vi "Autonomous Independent.vi"() -> ()   [LabVIEW 2011]
doc: "This VI is called when autonomous begins, and will automatically be terminated when autonomous ends. You can carry out timed or sensor driven robot movement independently without needing to return to the caller."
uses:
  Robot Global Data.vi
  <vilib>/addons/control/pid/pid.llb/PID (DBL).vi
  <vilib>/addons/control/pid/NI_PID_pid.lvlib
  <vilib>/Analysis/NI_AALBase.lvlib
panel:
  in  "Gains Left":T1={"proportional gain (Kc)"=0.01, "integral time (Ti, min)"=0.0, "derivative time (Td, min)"=0.001}
  in  "Gains Right":T1={"proportional gain (Kc)"=0.01, "integral time (Ti, min)"=0.0, "derivative time (Td, min)"=0.001}
  out "Right Output":dbl(graph)
  out "Right Encoder":dbl(graph)
  out "Left Enoder":dbl(graph)
  out "Left Output":dbl(graph)
  out "Autonomous Switch Value":dbl
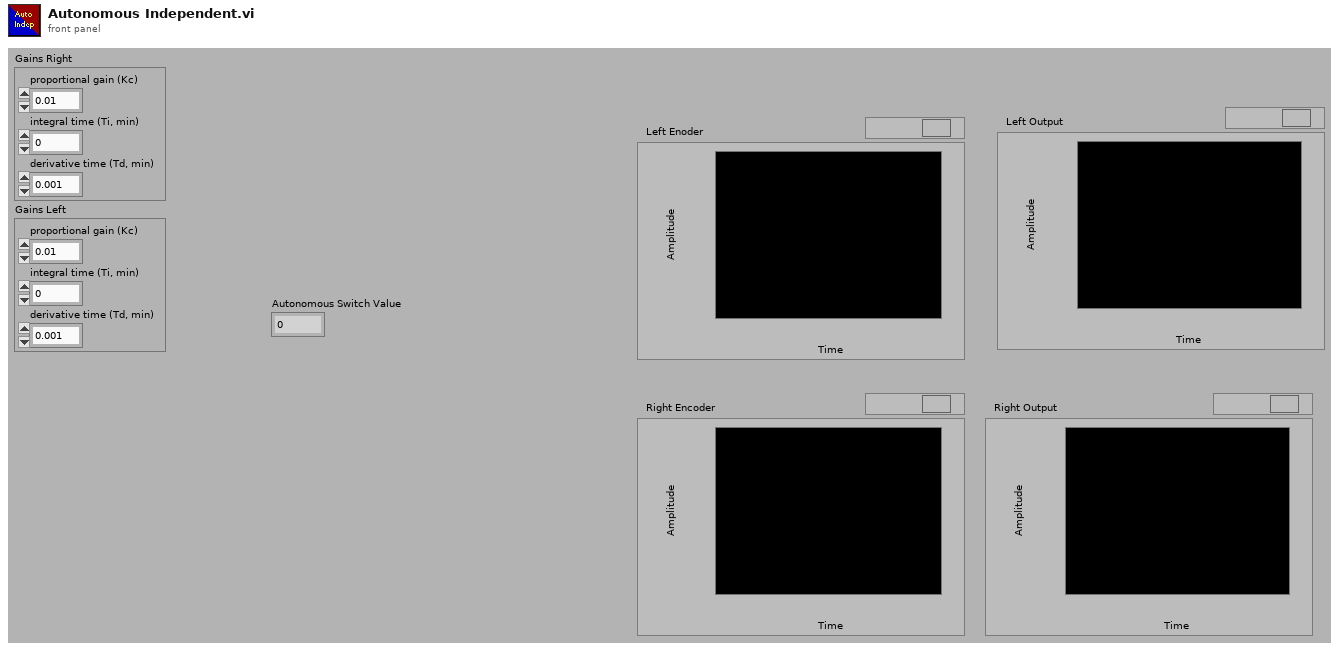
[diagram p1: front panel]
types:
  T1 = cluster{"proportional gain (Kc)":dbl, "integral time (Ti, min)":dbl, "derivative time (Td, min)":dbl}
  T2 = typedef "WPI_JoystickDevRef.ctl" = cluster{"Device":T3}
  T3 = typedef "WPI_JoystickDeviceEnum.ctl" = enum16{"USB 1", "USB 2", "USB 3", "USB 4", "Kinect 1", "Kinect 2"}
  T4 = typedef "WPI_DigitalInputDevRef.ctl" = cluster{"DevStatus":errorcluster, "DIO Channel":T5, "Digital Module":T6}
  T5 = typedef "FPGA_DIOChannel.ctl" = enum8{"DIO 1", "DIO 2", "DIO 3", "DIO 4", "DIO 5", "DIO 6", "DIO 7", "DIO 8", "DIO 9", "DIO 10", "DIO 11", "DIO 12", "DIO 13", "DIO 14", "Invalid"}
  T6 = typedef "FPGA_TypedefDigitalModule.ctl" = enum16{"Digital Module 1", "Digital Module 2"}
  T7 = cluster{"axis 1 (x)":dbl, "axis 2 (y)":dbl, "axis 3 (throttle)":dbl, "axis 4":dbl, "axis 5":dbl, "axis 6":dbl}
  T8 = enum16{"Shoot", "Load", "Arm", "Nothing", "Reverse", "ShootAll"}
  T9 = typedef "WPI_RobotDriveDevRef.ctl" = cluster{"DevStatus":errorcluster, "Motors[]":T10[], "Square Inputs":bool, "Max Output":dbl, "Isochronous":bool}
  T10 = typedef "WPI_MotorControlDeviceRef.ctl" = cluster{"DeviceStatus":errorcluster, "Type":enum16{"PWM", "CAN"}, "PWM":cluster{"Digital Module":T6, "PWM Channel":T11, "DeadBand":T12}, "CAN":cluster{"Device Number":u8, "Control Mode":T13, "Semaphore":T14, "Max Vout":dbl}, "Invert":bool, "TransformRef":T15, "InvTransformRef":T15}
  T11 = typedef "FPGA_DIOPWMChannel.ctl" = enum8{"PWM 1", "PWM 2", "PWM 3", "PWM 4", "PWM 5", "PWM 6", "PWM 7", "PWM 8", "PWM 9", "PWM 10", "Invalid"}
  T12 = typedef "WPI_PWMDeadband.ctl" = cluster{"Name":string, "maxPositivePwm":i32, "minPositivePwm":i32, "centerPwm":i32, "maxNegativePwm":i32, "minNegativePwm":i32, "angularRange":u16}
  T13 = typedef "WPI_CANJaguar_ControlMode.ctl" = enum8{"Percent VBus", "Current", "Speed", "Position", "Voltage"}
  T14 = typedef "Semaphore RefNum" = refnum<k1>
  T15 = typedef "WPI_PWMTransform_ConPane.ctl" = refnum<vi>
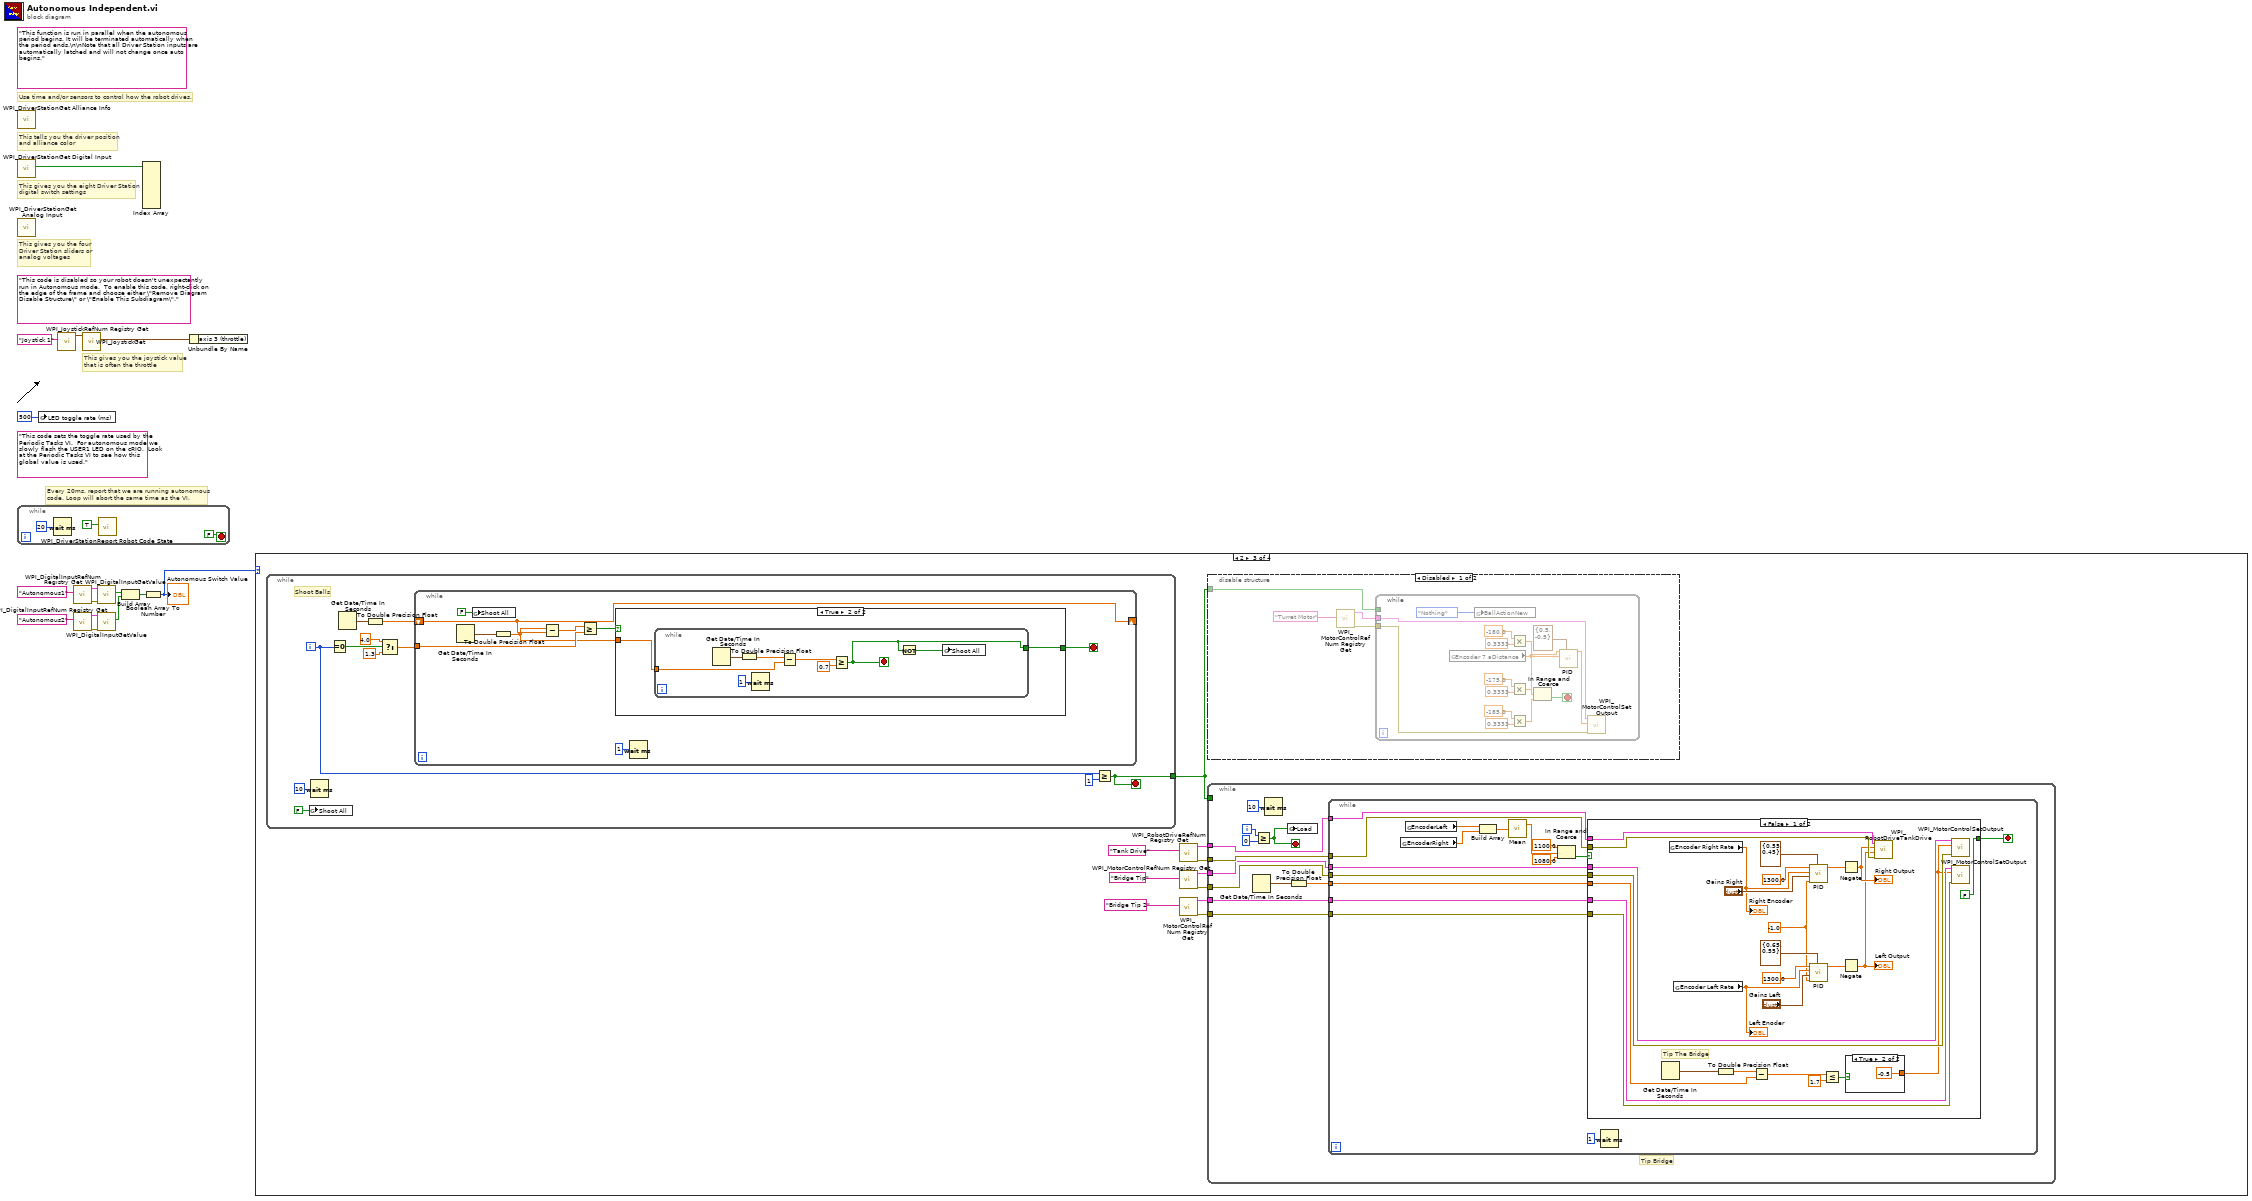
[diagram p0: block diagram]
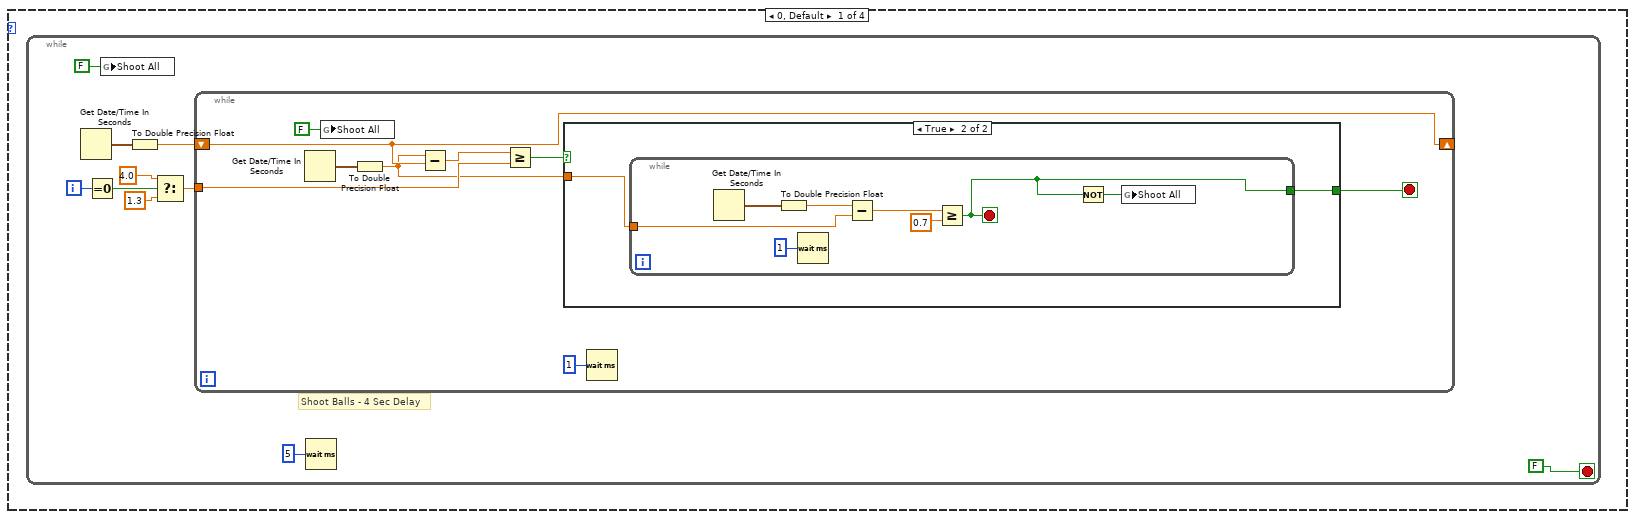
[diagram p2: hidden frame]
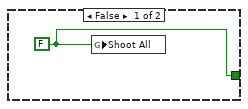
[diagram p3: hidden frame]
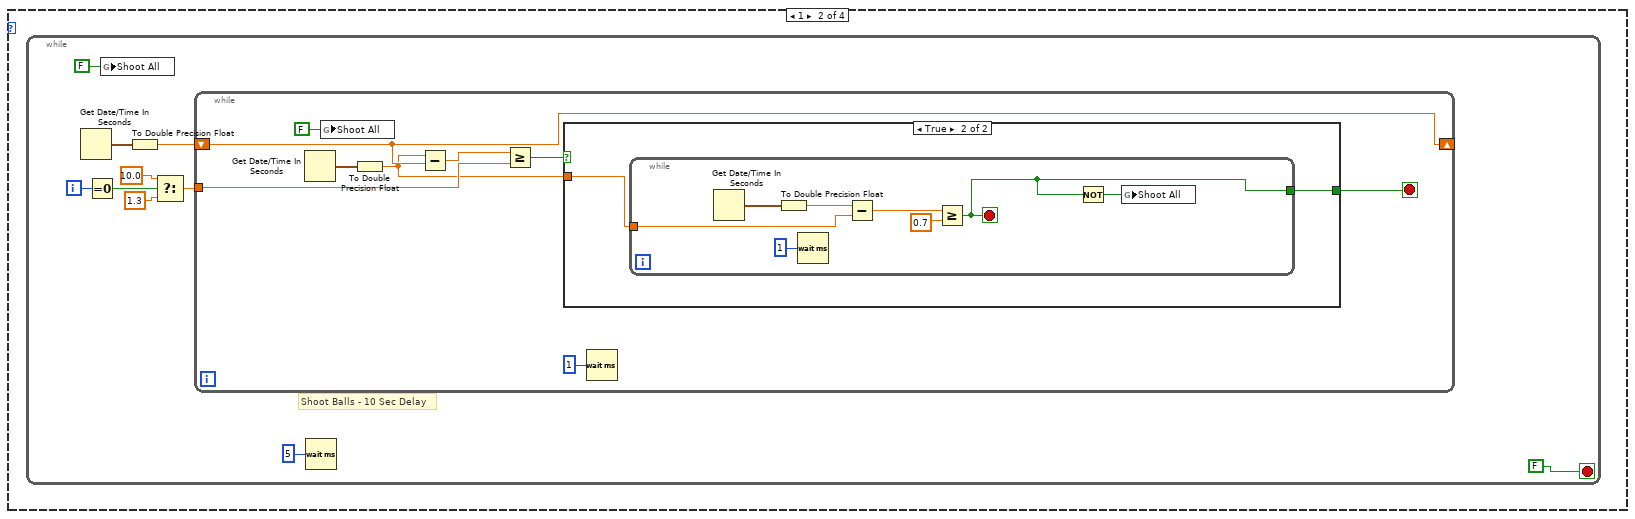
[diagram p4: hidden frame]
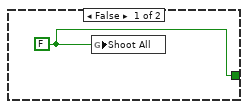
[diagram p5: hidden frame]
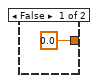
[diagram p7: hidden frame]
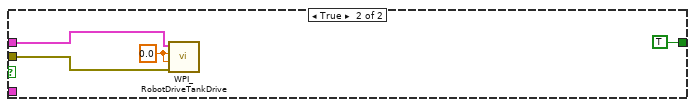
[diagram p8: hidden frame]
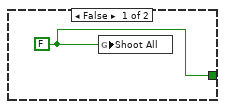
[diagram p9: hidden frame]
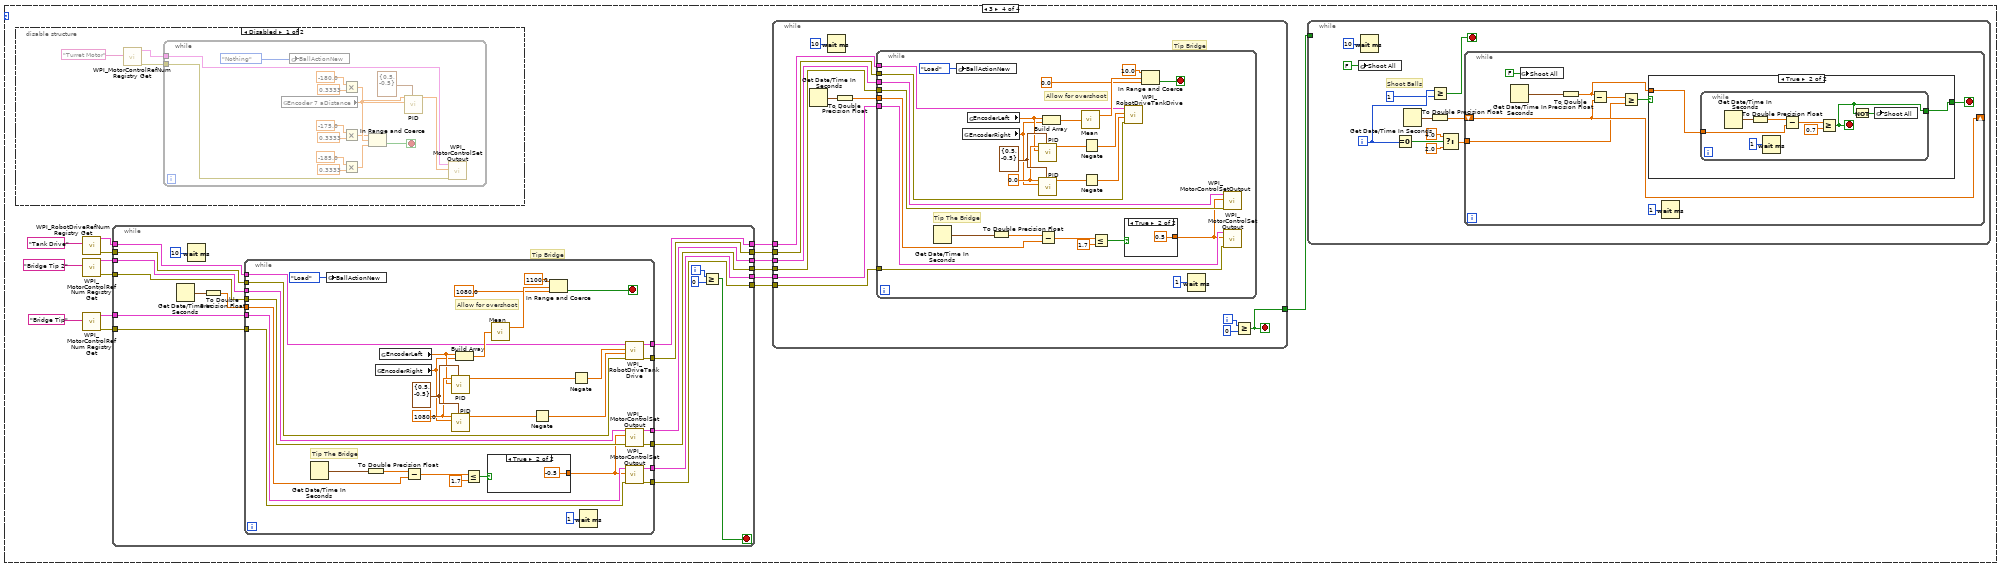
[diagram p10: hidden frame]
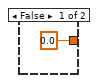
[diagram p11: hidden frame]
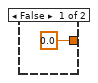
[diagram p13: hidden frame]
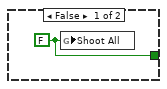
[diagram p14: hidden frame]
diagram:
  (unwired) "This code sets the toggle rate used by the Periodic Tasks VI.  For autonomous mode we slowly flash the USER1 LED on the cRIO.  Look at the Periodic Tasks VI to see how this global value is used."
  (unwired) "This code is disabled so your robot doesn't unexpectantly run in Autonomous mode.  To enable this code, right-click on the edge of the frame and choose either \"Remove Diagram Disable Structure\" or \"Enable This Subdiagram\"."
  (unwired) "This function is run in parallel when the autonomous period begins. It will be terminated automatically when the period ends.\n\nNote that all Driver Station inputs are automatically latched and will not change once auto begins."
  # "Every 20ms, report that we are running autonomous\ncode. Loop will abort the same time as the VI."
  # "This gives you the joystick value\nthat is often the throttle"
  # "Use time and/or sensors to control how the robot drives."
  # "This tells you the driver position\nand alliance color"
  # "This gives you the eight Driver Station\ndigital switch settings"
  # "This gives you the four\nDriver Station sliders or\nanalog voltages"
  n1 = call <vilib>:"WPI_DriverStationGet Alliance Info.vi"() -> ()  [unwired: 12 out]
  n2 = call <vilib>:"WPI_DriverStationGet Digital Input.vi"() -> ("Driver Station Digital Input (1-8)"=w15:bool[])  [unwired: 11 out]
  n3 = call <vilib>:"WPI_DriverStationGet Analog Input.vi"() -> ()  [unwired: 12 out]
  n4 = while {
    stop <- FALSE stop-if-true
    n5 = Wait (ms)(milliseconds to wait=u32 20) -> ()  [unwired: 1 out]
    n6 = call <vilib>:"WPI_DriverStationReport Robot Code State.vi"("Autonomous"=TRUE) -> ()  [unwired: 10 in, 1 out]
  }
  n7 = global write "Robot Global Data.vi" "LED toggle rate (ms)"(u32 500 ("LED ms toggle rate")) -> ()
  n8 = call <vilib>:"WPI_JoystickRefNum Registry Get.vi"("refnum name"="Joystick 1") -> ("JoystickDevRef"=w12:T2)  [unwired: 1 in, 9 out]
  n9 = call <vilib>:"WPI_DigitalInputRefNum Registry Get.vi"("refnum name"="Autonomous1") -> ("error out"=w8:errorcluster, "DigitalInputDevRef"=w7:T4)  [unwired: 9 in]
  n10 = call <vilib>:"WPI_DigitalInputRefNum Registry Get.vi"("refnum name"="Autonomous2") -> ("error out"=w5:errorcluster, "DigitalInputDevRef"=w6:T4)  [unwired: 9 in]
  n11 = call <vilib>:"WPI_JoystickGet.vi"("JoystickDevRef"=w12) -> ("Axes"=w13:T7)  [unwired: 1 in, 5 out]
  n12 = call <vilib>:"WPI_DigitalInputGetValue.vi"("error in (no error)"=w8, "DigitalInputDevRef"=w7) -> ("Value"=w9:bool)  [unwired: 7 in, 2 out]
  n13 = call <vilib>:"WPI_DigitalInputGetValue.vi"("error in (no error)"=w5, "DigitalInputDevRef"=w6) -> ("Value"=w10:bool)  [unwired: 7 in, 2 out]
  n14 = Build Array(w9, w10) -> (w2:bool[])
  n15 = Index Array(array=w15) -> ()  [unwired: 8 in, 8 out]
  n16 = Boolean Array To Number(Boolean array=w2) -> (number=w1:u32)
  "Autonomous Switch Value" <- w1
  n17 = Unbundle By Name(w13) -> ()  [unwired: 1 out]
  n18 = case shown="2" w1 {
    frame 0, Default {
      n19 = while {
        i -> [w24]
        stop <- FALSE stop-if-true
        # "Shoot Balls - 4 Sec Delay"
        n20 = Get Date/Time In Seconds() -> (seconds since 1Jan1904=w28:timestamp)
        n21 = Equal To 0?(x=w24) -> (x = 0?=w23:bool)
        n22 = global write "Robot Global Data.vi" "Shoot All"(FALSE ("Shoot All")) -> ()
        n23 = To Double Precision Float(number=w28) -> (double precision float=w27:dbl)
        n24 = Select(t=4.0, s=w23, f=1.3) -> (s? t:f=w22:dbl)
        n25 = while {
          shift-right: [w37] -> _
          shift-left: w27 -> [w37]
          tunnel: w22 -> [w35]
          stop <- w34 stop-if-true
          n26 = Get Date/Time In Seconds() -> (seconds since 1Jan1904=w33:timestamp)
          n27 = global write "Robot Global Data.vi" "Shoot All"(FALSE ("Shoot All")) -> ()
          n28 = To Double Precision Float(number=w33) -> (double precision float=w31:dbl)
          n29 = Subtract(x=w31, y=w37) -> (x-y=w32:dbl)
          n30 = Greater Or Equal?(x=w32, y=w35) -> (x >= y?=w30:bool)
          n31 = case shown="True" w30 {
            tunnel: [w38 w40] -> w34
            tunnel: w31 -> [_ w39]
            frame False {
              w38 = FALSE
              n32 = global write "Robot Global Data.vi" "Shoot All"(w38) -> ()
            }
            frame True {
              n33 = while {
                tunnel: w39 -> [w46]
                tunnel: [w41] -> w40
                stop <- w41 stop-if-true
                n34 = Get Date/Time In Seconds() -> (seconds since 1Jan1904=w48:timestamp)
                n35 = To Double Precision Float(number=w48) -> (double precision float=w47:dbl)
                n36 = Wait (ms)(milliseconds to wait=u32 1) -> ()  [unwired: 1 out]
                n37 = Subtract(x=w47, y=w46) -> (x-y=w45:dbl)
                n38 = Greater Or Equal?(x=w45, y=0.7) -> (x >= y?=w41:bool)
                n39 = Not(x=w41) -> (.not. x?=w42:bool)
                n40 = global write "Robot Global Data.vi" "Shoot All"(w42) -> ()
              }
            }
          }
          n41 = Wait (ms)(milliseconds to wait=u32 1) -> ()  [unwired: 1 out]
        }
        n42 = Wait (ms)(milliseconds to wait=u32 5) -> ()  [unwired: 1 out]
      }
    }
    frame 1 {
      n43 = while {
        i -> [w54]
        stop <- FALSE stop-if-true
        # "Shoot Balls - 10 Sec Delay"
        n44 = Get Date/Time In Seconds() -> (seconds since 1Jan1904=w58:timestamp)
        n45 = Equal To 0?(x=w54) -> (x = 0?=w53:bool)
        n46 = global write "Robot Global Data.vi" "Shoot All"(FALSE ("Shoot All")) -> ()
        n47 = To Double Precision Float(number=w58) -> (double precision float=w57:dbl)
        n48 = Select(t=10.0, s=w53, f=1.3) -> (s? t:f=w52:dbl)
        n49 = while {
          shift-right: [w67] -> _
          shift-left: w57 -> [w67]
          tunnel: w52 -> [w65]
          stop <- w64 stop-if-true
          n50 = Get Date/Time In Seconds() -> (seconds since 1Jan1904=w63:timestamp)
          n51 = global write "Robot Global Data.vi" "Shoot All"(FALSE ("Shoot All")) -> ()
          n52 = To Double Precision Float(number=w63) -> (double precision float=w61:dbl)
          n53 = Subtract(x=w61, y=w67) -> (x-y=w62:dbl)
          n54 = Greater Or Equal?(x=w62, y=w65) -> (x >= y?=w60:bool)
          n55 = case shown="True" w60 {
            tunnel: [w68 w70] -> w64
            tunnel: w61 -> [_ w69]
            frame False {
              w68 = FALSE
              n56 = global write "Robot Global Data.vi" "Shoot All"(w68) -> ()
            }
            frame True {
              n57 = while {
                tunnel: w69 -> [w76]
                tunnel: [w71] -> w70
                stop <- w71 stop-if-true
                n58 = Get Date/Time In Seconds() -> (seconds since 1Jan1904=w78:timestamp)
                n59 = To Double Precision Float(number=w78) -> (double precision float=w77:dbl)
                n60 = Wait (ms)(milliseconds to wait=u32 1) -> ()  [unwired: 1 out]
                n61 = Subtract(x=w77, y=w76) -> (x-y=w75:dbl)
                n62 = Greater Or Equal?(x=w75, y=0.7) -> (x >= y?=w71:bool)
                n63 = Not(x=w71) -> (.not. x?=w72:bool)
                n64 = global write "Robot Global Data.vi" "Shoot All"(w72) -> ()
              }
            }
          }
          n65 = Wait (ms)(milliseconds to wait=u32 1) -> ()  [unwired: 1 out]
        }
        n66 = Wait (ms)(milliseconds to wait=u32 5) -> ()  [unwired: 1 out]
      }
    }
    frame 2 {
      n67 = while {
        tunnel: [w170] -> w79
        i -> [w172]
        stop <- w170 stop-if-true
        # "Shoot Balls"
        n68 = global write "Robot Global Data.vi" "Shoot All"(FALSE ("Shoot All")) -> ()
        n69 = Wait (ms)(milliseconds to wait=u32 10) -> ()  [unwired: 1 out]
        n70 = Equal To 0?(x=w172) -> (x = 0?=w177:bool)
        n71 = Get Date/Time In Seconds() -> (seconds since 1Jan1904=w180:timestamp)
        n72 = To Double Precision Float(number=w180) -> (double precision float=w179:dbl)
        n73 = Select(t=4.0, s=w177, f=1.3) -> (s? t:f=w176:dbl)
        n74 = while {
          shift-right: [w189] -> _
          shift-left: w179 -> [w189]
          tunnel: w176 -> [w187]
          stop <- w186 stop-if-true
          n75 = Get Date/Time In Seconds() -> (seconds since 1Jan1904=w185:timestamp)
          n76 = global write "Robot Global Data.vi" "Shoot All"(FALSE ("Shoot All")) -> ()
          n77 = To Double Precision Float(number=w185) -> (double precision float=w183:dbl)
          n78 = Subtract(x=w183, y=w189) -> (x-y=w184:dbl)
          n79 = Greater Or Equal?(x=w184, y=w187) -> (x >= y?=w182:bool)
          n80 = case shown="True" w182 {
            tunnel: [w190 w192] -> w186
            tunnel: w183 -> [_ w191]
            frame False {
              w190 = FALSE
              n81 = global write "Robot Global Data.vi" "Shoot All"(w190) -> ()
            }
            frame True {
              n82 = while {
                tunnel: w191 -> [w198]
                tunnel: [w193] -> w192
                stop <- w193 stop-if-true
                n83 = Get Date/Time In Seconds() -> (seconds since 1Jan1904=w200:timestamp)
                n84 = To Double Precision Float(number=w200) -> (double precision float=w199:dbl)
                n85 = Wait (ms)(milliseconds to wait=u32 1) -> ()  [unwired: 1 out]
                n86 = Subtract(x=w199, y=w198) -> (x-y=w197:dbl)
                n87 = Greater Or Equal?(x=w197, y=0.7) -> (x >= y?=w193:bool)
                n88 = Not(x=w193) -> (.not. x?=w194:bool)
                n89 = global write "Robot Global Data.vi" "Shoot All"(w194) -> ()
              }
            }
          }
          n90 = Wait (ms)(milliseconds to wait=u32 1) -> ()  [unwired: 1 out]
        }
        n91 = Greater Or Equal?(x=w172, y=1) -> (x >= y?=w170:bool)
      }
      n92 = call <vilib>:"WPI_RobotDriveRefNum Registry Get.vi"("refnum name"="Tank Drive") -> ("error out"=w80:errorcluster, "RobotDriveDevRef"=w81:T9)  [unwired: 9 in]
      n93 = call <vilib>:"WPI_MotorControlRefNum Registry Get.vi"("refnum name"="Bridge Tip") -> ("error out"=w85:errorcluster, "MotorControlDevRef"=w86:T10)  [unwired: 9 in]
      n94 = call <vilib>:"WPI_MotorControlRefNum Registry Get.vi"("refnum name"="Bridge Tip 2") -> ("error out"=w83:errorcluster, "MotorControlDevRef"=w84:T10)  [unwired: 9 in]
      n95 = disable-structure shown="Disabled" {
        disable-tunnel: w79 -> [w92 _]
        frame Disabled {
          n96 = call <vilib>:"WPI_MotorControlRefNum Registry Get.vi"("refnum name"="Turret Motor") -> ("error out"=w89:errorcluster, "MotorControlDevRef"=w90:T10)  [unwired: 9 in]
          n97 = while {
            tunnel: w92 -> [_]
            tunnel: w90 -> [w104]
            tunnel: w89 -> [w103]
            stop <- w93 stop-if-true
            n98 = global read "Robot Global Data.vi" "Encoder 7 aDistance"() -> (w105:dbl)
            n99 = global write "Robot Global Data.vi" "BallActionNew"(T8."Nothing" ("BallActionNew")) -> ()
            n100 = Multiply(x=-180.0, y=0.3333) -> (x*y=w101:dbl)
            n101 = Multiply(x=-175.0, y=0.3333) -> (x*y=w96:dbl)
            n102 = Multiply(x=-185.0, y=0.3333) -> (x*y=w95:dbl)
            n103 = In Range and Coerce(upper limit=w96, x=w105, lower limit=w95) -> (In Range?=w93:bool)  [unwired: 1 out]
            n104 = call-poly <vilib>:"PID.vi"("output range"=cluster{"output high":dbl, "output low":dbl} {"output high"=0.5, "output low"=-0.5}, "process variable"=w105, "setpoint"=w101) -> ("output"=w107:dbl)  [unwired: 7 in, 1 out]
            n105 = call <vilib>:"WPI_MotorControlSetOutput.vi"("error in (no error)"=w103, "Output"=w107, "MotorControlDevRef"=w104) -> ()  [unwired: 7 in, 2 out]
          }
        }
        frame Enabled {
        }
      }
      n106 = while {
        tunnel: w86 -> [w111]
        tunnel: w85 -> [w112]
        tunnel: w84 -> [w114]
        tunnel: w83 -> [w115]
        tunnel: w81 -> [w116]
        tunnel: w80 -> [w117]
        tunnel: w79 -> [_]
        i -> [w110]
        stop <- w109 stop-if-true
        # "Tip Bridge"
        n107 = Get Date/Time In Seconds() -> (seconds since 1Jan1904=w120:timestamp)
        n108 = Greater Or Equal?(x=w110, y=0) -> (x >= y?=w109:bool)
        n109 = Wait (ms)(milliseconds to wait=u32 10) -> ()  [unwired: 1 out]
        n110 = global write "Robot Global Data.vi" "Load"(w109) -> ()
        n111 = To Double Precision Float(number=w120) -> (double precision float=w113:dbl)
        n112 = while {
          tunnel: w111 -> [w130]
          tunnel: w112 -> [w129]
          tunnel: w114 -> [w132]
          tunnel: w115 -> [w131]
          tunnel: w116 -> [w135]
          tunnel: w117 -> [w134]
          tunnel: w113 -> [w133]
          stop <- w121 stop-if-true
          n113 = global read "Robot Global Data.vi" "EncoderRight"() -> (w128:dbl)
          n114 = global read "Robot Global Data.vi" "EncoderLeft"() -> (w127:dbl)
          n115 = Build Array(w127, w128) -> (w126:dbl[])
          n116 = call <vilib>:"Mean.vi"("X"=w126) -> ("mean"=w124:dbl)  [unwired: 1 out]
          n117 = In Range and Coerce(upper limit=1100.0, x=w124, lower limit=1080.0) -> (In Range?=w122:bool)  [unwired: 1 out]
          n118 = case shown="False" w122 {
            tunnel: w135 -> [w151 w168]
            tunnel: w134 -> [w150 w167]
            tunnel: w133 -> [w161 _]
            tunnel: w132 -> [w157 _]
            tunnel: w131 -> [w156 _]
            tunnel: w130 -> [w155 _]
            tunnel: w129 -> [w154 _]
            tunnel: [FALSE TRUE] -> w121
            frame False {
              w140 = -1.0 ("dt (s)")
              # "Tip The Bridge"
              n119 = Get Date/Time In Seconds() -> (seconds since 1Jan1904=w163:timestamp)
              n120 = global read "Robot Global Data.vi" "Encoder Right Rate"() -> (w143:dbl)
              "Right Encoder" <- w143
              n121 = global read "Robot Global Data.vi" "Encoder Left Rate"() -> (w142:dbl)
              "Left Enoder" <- w142
              n122 = To Double Precision Float(number=w163) -> (double precision float=w162:dbl)
              n123 = Subtract(x=w162, y=w161) -> (x-y=w159:dbl)
              n124 = call-poly <vilib>:"PID.vi"("output range"=cluster{"output high":dbl, "output low":dbl} {"output high"=0.55, "output low"=0.45}, "dt (s)"=w140, "PID gains"="Gains Right", "process variable"=w143, "setpoint"=1300.0 ("lower limit")) -> ("output"=w144:dbl)  [unwired: 5 in, 1 out]
              n125 = call-poly <vilib>:"PID.vi"("output range"=cluster{"output high":dbl, "output low":dbl} {"output high"=0.65, "output low"=0.55}, "dt (s)"=w140, "PID gains"="Gains Left", "process variable"=w142, "setpoint"=1300.0 ("lower limit")) -> ("output"=w148:dbl)  [unwired: 5 in, 1 out]
              n126 = Less Or Equal?(x=w159, y=1.7) -> (x <= y?=w160:bool)
              n127 = Negate(x=w144) -> (-x=w138:dbl)
              "Right Output" <- w138
              n128 = Negate(x=w148) -> (-x=w137:dbl)
              "Left Output" <- w137
              n129 = case shown="True" w160 {
                tunnel: [0.0 ("Output") -0.5 ("Output")] -> w153
                frame False {
                }
                frame True {
                }
              }
              n130 = call <vilib>:"WPI_RobotDriveTankDrive.vi"("error in (no error)"=w150, "Right axis value"=w137, "Left axis value"=w138, "RobotDriveDevRef"=w151) -> ()  [unwired: 6 in, 2 out]
              n131 = call <vilib>:"WPI_MotorControlSetOutput.vi"("error in (no error)"=w154, "Output"=w153, "MotorControlDevRef"=w155) -> ()  [unwired: 7 in, 2 out]
              n132 = call <vilib>:"WPI_MotorControlSetOutput.vi"("error in (no error)"=w156, "Output"=w153, "MotorControlDevRef"=w157) -> ()  [unwired: 7 in, 2 out]
            }
            frame True {
              w166 = 0.0 ("Right axis value")
              n133 = call <vilib>:"WPI_RobotDriveTankDrive.vi"("error in (no error)"=w167, "Right axis value"=w166, "Left axis value"=w166, "RobotDriveDevRef"=w168) -> ()  [unwired: 6 in, 2 out]
            }
          }
          n134 = Wait (ms)(milliseconds to wait=u32 1) -> ()  [unwired: 1 out]
        }
      }
    }
    frame 3 {
      n135 = disable-structure shown="Disabled" {
        frame Disabled {
          n136 = call <vilib>:"WPI_MotorControlRefNum Registry Get.vi"("refnum name"="Turret Motor") -> ("error out"=w259:errorcluster, "MotorControlDevRef"=w260:T10)  [unwired: 9 in]
          n137 = while {
            tunnel: w260 -> [w272]
            tunnel: w259 -> [w271]
            stop <- w273 stop-if-true
            n138 = global read "Robot Global Data.vi" "Encoder 7 aDistance"() -> (w274:dbl)
            n139 = global write "Robot Global Data.vi" "BallActionNew"(T8."Nothing" ("BallActionNew")) -> ()
            n140 = Multiply(x=-180.0, y=0.3333) -> (x*y=w269:dbl)
            n141 = Multiply(x=-175.0, y=0.3333) -> (x*y=w264:dbl)
            n142 = Multiply(x=-185.0, y=0.3333) -> (x*y=w263:dbl)
            n143 = In Range and Coerce(upper limit=w264, x=w274, lower limit=w263) -> (In Range?=w273:bool)  [unwired: 1 out]
            n144 = call-poly <vilib>:"PID.vi"("output range"=cluster{"output high":dbl, "output low":dbl} {"output high"=0.5, "output low"=-0.5}, "process variable"=w274, "setpoint"=w269) -> ("output"=w276:dbl)  [unwired: 7 in, 1 out]
            n145 = call <vilib>:"WPI_MotorControlSetOutput.vi"("error in (no error)"=w271, "Output"=w276, "MotorControlDevRef"=w272) -> ()  [unwired: 7 in, 2 out]
          }
        }
        frame Enabled {
        }
      }
      n146 = call <vilib>:"WPI_RobotDriveRefNum Registry Get.vi"("refnum name"="Tank Drive") -> ("error out"=w208:errorcluster, "RobotDriveDevRef"=w209:T9)  [unwired: 9 in]
      n147 = call <vilib>:"WPI_MotorControlRefNum Registry Get.vi"("refnum name"="Bridge Tip 2") -> ("error out"=w211:errorcluster, "MotorControlDevRef"=w212:T10)  [unwired: 9 in]
      n148 = call <vilib>:"WPI_MotorControlRefNum Registry Get.vi"("refnum name"="Bridge Tip") -> ("error out"=w213:errorcluster, "MotorControlDevRef"=w214:T10)  [unwired: 9 in]
      n149 = while {
        tunnel: w214 -> [w295]
        tunnel: w213 -> [w294]
        tunnel: w212 -> [w293]
        tunnel: w211 -> [w292]
        tunnel: w209 -> [w291]
        tunnel: w208 -> [w290]
        tunnel: [w283] -> w207
        tunnel: [w282] -> w206
        tunnel: [w281] -> w205
        tunnel: [w280] -> w204
        tunnel: [w279] -> w203
        tunnel: [w278] -> w202
        i -> [w286]
        stop <- w284 stop-if-true
        # "Tip Bridge"
        n150 = Get Date/Time In Seconds() -> (seconds since 1Jan1904=w289:timestamp)
        n151 = Wait (ms)(milliseconds to wait=u32 10) -> ()  [unwired: 1 out]
        n152 = To Double Precision Float(number=w289) -> (double precision float=w288:dbl)
        n153 = while {
          tunnel: w295 -> [w311]
          tunnel: w294 -> [w310]
          tunnel: w293 -> [w313]
          tunnel: w292 -> [w312]
          tunnel: w291 -> [w323]
          tunnel: w290 -> [w322]
          tunnel: w288 -> [w317]
          tunnel: [w301] -> w283
          tunnel: [w300] -> w282
          tunnel: [w299] -> w281
          tunnel: [w298] -> w280
          tunnel: [w297] -> w279
          tunnel: [w296] -> w278
          stop <- w328 stop-if-true
          w308 = cluster{"output high":dbl, "output low":dbl} {"output high"=0.5, "output low"=-0.5} ("output range")
          w307 = 1080.0 ("setpoint")
          # "Allow for overshoot"
          # "Tip The Bridge"
          n154 = Get Date/Time In Seconds() -> (seconds since 1Jan1904=w319:timestamp)
          n155 = global write "Robot Global Data.vi" "BallActionNew"(T8."Load" ("BallActionNew")) -> ()
          n156 = To Double Precision Float(number=w319) -> (double precision float=w318:dbl)
          n157 = global read "Robot Global Data.vi" "EncoderRight"() -> (w304:dbl)
          n158 = global read "Robot Global Data.vi" "EncoderLeft"() -> (w305:dbl)
          n159 = Subtract(x=w318, y=w317) -> (x-y=w315:dbl)
          n160 = call-poly <vilib>:"PID.vi"("output range"=w308, "process variable"=w305, "setpoint"=w307) -> ("output"=w306:dbl)  [unwired: 7 in, 1 out]
          n161 = call-poly <vilib>:"PID.vi"("output range"=w308, "process variable"=w304, "setpoint"=w307) -> ("output"=w320:dbl)  [unwired: 7 in, 1 out]
          n162 = Build Array(w305, w304) -> (w329:dbl[])
          n163 = Less Or Equal?(x=w315, y=1.7) -> (x <= y?=w316:bool)
          n164 = case shown="True" w316 {
            tunnel: [0.0 ("Output") -0.5 ("Output")] -> w309
            frame False {
            }
            frame True {
            }
          }
          n165 = call <vilib>:"Mean.vi"("X"=w329) -> ("mean"=w327:dbl)  [unwired: 1 out]
          n166 = Negate(x=w320) -> (-x=w302:dbl)
          n167 = In Range and Coerce(upper limit=1100.0, x=w327, lower limit=1080.0) -> (In Range?=w328:bool)  [unwired: 1 out]
          n168 = Negate(x=w306) -> (-x=w303:dbl)
          n169 = Wait (ms)(milliseconds to wait=u32 1) -> ()  [unwired: 1 out]
          n170 = call <vilib>:"WPI_RobotDriveTankDrive.vi"("error in (no error)"=w322, "Right axis value"=w302, "Left axis value"=w303, "RobotDriveDevRef"=w323) -> ("error out"=w300:errorcluster, "RobotDriveDevRef"=w301:T9)  [unwired: 6 in]
          n171 = call <vilib>:"WPI_MotorControlSetOutput.vi"("error in (no error)"=w312, "Output"=w309, "MotorControlDevRef"=w313) -> ("error out"=w296:errorcluster, "MotorControlDevRef"=w297:T10)  [unwired: 7 in]
          n172 = call <vilib>:"WPI_MotorControlSetOutput.vi"("error in (no error)"=w310, "Output"=w309, "MotorControlDevRef"=w311) -> ("error out"=w298:errorcluster, "MotorControlDevRef"=w299:T10)  [unwired: 7 in]
        }
        n173 = Greater Or Equal?(x=w286, y=0) -> (x >= y?=w284:bool)
      }
      n174 = while {
        tunnel: w205 -> [w228]
        tunnel: w204 -> [w227]
        tunnel: w203 -> [w226]
        tunnel: w202 -> [w225]
        tunnel: w207 -> [w224]
        tunnel: w206 -> [w223]
        tunnel: [w217] -> w201
        i -> [w219]
        stop <- w217 stop-if-true
        # "Tip Bridge"
        n175 = Get Date/Time In Seconds() -> (seconds since 1Jan1904=w222:timestamp)
        n176 = Wait (ms)(milliseconds to wait=u32 10) -> ()  [unwired: 1 out]
        n177 = To Double Precision Float(number=w222) -> (double precision float=w221:dbl)
        n178 = while {
          tunnel: w228 -> [w238]
          tunnel: w227 -> [w237]
          tunnel: w226 -> [w240]
          tunnel: w225 -> [w239]
          tunnel: w224 -> [w250]
          tunnel: w223 -> [w249]
          tunnel: w221 -> [w244]
          stop <- w255 stop-if-true
          w235 = cluster{"output high":dbl, "output low":dbl} {"output high"=0.5, "output low"=-0.5} ("output range")
          w234 = 0.0 ("setpoint")
          # "Allow for overshoot"
          # "Tip The Bridge"
          n179 = Get Date/Time In Seconds() -> (seconds since 1Jan1904=w246:timestamp)
          n180 = global write "Robot Global Data.vi" "BallActionNew"(T8."Load" ("BallActionNew")) -> ()
          n181 = global read "Robot Global Data.vi" "EncoderRight"() -> (w231:dbl)
          n182 = global read "Robot Global Data.vi" "EncoderLeft"() -> (w232:dbl)
          n183 = To Double Precision Float(number=w246) -> (double precision float=w245:dbl)
          n184 = call-poly <vilib>:"PID.vi"("output range"=w235, "process variable"=w232, "setpoint"=w234) -> ("output"=w233:dbl)  [unwired: 7 in, 1 out]
          n185 = call-poly <vilib>:"PID.vi"("output range"=w235, "process variable"=w231, "setpoint"=w234) -> ("output"=w247:dbl)  [unwired: 7 in, 1 out]
          n186 = Subtract(x=w245, y=w244) -> (x-y=w242:dbl)
          n187 = Build Array(w232, w231) -> (w256:dbl[])
          n188 = call <vilib>:"Mean.vi"("X"=w256) -> ("mean"=w254:dbl)  [unwired: 1 out]
          n189 = Negate(x=w233) -> (-x=w230:dbl)
          n190 = Negate(x=w247) -> (-x=w229:dbl)
          n191 = Less Or Equal?(x=w242, y=1.7) -> (x <= y?=w243:bool)
          n192 = call <vilib>:"WPI_RobotDriveTankDrive.vi"("error in (no error)"=w249, "Right axis value"=w229, "Left axis value"=w230, "RobotDriveDevRef"=w250) -> ()  [unwired: 6 in, 2 out]
          n193 = case shown="True" w243 {
            tunnel: [0.0 ("Output") 0.5 ("Output")] -> w236
            frame False {
            }
            frame True {
            }
          }
          n194 = In Range and Coerce(upper limit=10.0, x=w254, lower limit=0.0) -> (In Range?=w255:bool)  [unwired: 1 out]
          n195 = Wait (ms)(milliseconds to wait=u32 1) -> ()  [unwired: 1 out]
          n196 = call <vilib>:"WPI_MotorControlSetOutput.vi"("error in (no error)"=w239, "Output"=w236, "MotorControlDevRef"=w240) -> ()  [unwired: 7 in, 2 out]
          n197 = call <vilib>:"WPI_MotorControlSetOutput.vi"("error in (no error)"=w237, "Output"=w236, "MotorControlDevRef"=w238) -> ()  [unwired: 7 in, 2 out]
        }
        n198 = Greater Or Equal?(x=w219, y=0) -> (x >= y?=w217:bool)
      }
      n199 = while {
        tunnel: w201 -> [_]
        i -> [w334]
        stop <- w332 stop-if-true
        # "Shoot Balls"
        n200 = global write "Robot Global Data.vi" "Shoot All"(FALSE ("Shoot All")) -> ()
        n201 = Wait (ms)(milliseconds to wait=u32 10) -> ()  [unwired: 1 out]
        n202 = Equal To 0?(x=w334) -> (x = 0?=w339:bool)
        n203 = Get Date/Time In Seconds() -> (seconds since 1Jan1904=w342:timestamp)
        n204 = To Double Precision Float(number=w342) -> (double precision float=w341:dbl)
        n205 = Greater Or Equal?(x=w334, y=1) -> (x >= y?=w332:bool)
        n206 = Select(t=4.0, s=w339, f=2.0) -> (s? t:f=w338:dbl)
        n207 = while {
          shift-right: [w351] -> _
          shift-left: w341 -> [w351]
          tunnel: w338 -> [w349]
          stop <- w348 stop-if-true
          n208 = Get Date/Time In Seconds() -> (seconds since 1Jan1904=w347:timestamp)
          n209 = global write "Robot Global Data.vi" "Shoot All"(FALSE ("Shoot All")) -> ()
          n210 = To Double Precision Float(number=w347) -> (double precision float=w345:dbl)
          n211 = Subtract(x=w345, y=w351) -> (x-y=w346:dbl)
          n212 = Greater Or Equal?(x=w346, y=w349) -> (x >= y?=w344:bool)
          n213 = case shown="True" w344 {
            tunnel: [w352 w354] -> w348
            tunnel: w345 -> [_ w353]
            frame False {
              w352 = FALSE
              n214 = global write "Robot Global Data.vi" "Shoot All"(w352) -> ()
            }
            frame True {
              n215 = while {
                tunnel: w353 -> [w360]
                tunnel: [w355] -> w354
                stop <- w355 stop-if-true
                n216 = Get Date/Time In Seconds() -> (seconds since 1Jan1904=w362:timestamp)
                n217 = To Double Precision Float(number=w362) -> (double precision float=w361:dbl)
                n218 = Wait (ms)(milliseconds to wait=u32 1) -> ()  [unwired: 1 out]
                n219 = Subtract(x=w361, y=w360) -> (x-y=w359:dbl)
                n220 = Greater Or Equal?(x=w359, y=0.7) -> (x >= y?=w355:bool)
                n221 = Not(x=w355) -> (.not. x?=w356:bool)
                n222 = global write "Robot Global Data.vi" "Shoot All"(w356) -> ()
              }
            }
          }
          n223 = Wait (ms)(milliseconds to wait=u32 1) -> ()  [unwired: 1 out]
        }
      }
    }
  }
